vi "LINC Register COSMOS Commands.vi"(8 "error in":errorcluster, 11 "LINC session":refnum<class "LINC.lvclass">) -> (0 "error out":errorcluster, 3 "dup LINC session":refnum<class "LINC.lvclass">)   [LabVIEW 2018, in "STEPkgDriver_LINC.lvlib" / "LINC.lvclass"]
uses:
  LINC.lvclass
panel:
  in  "common commands":T1
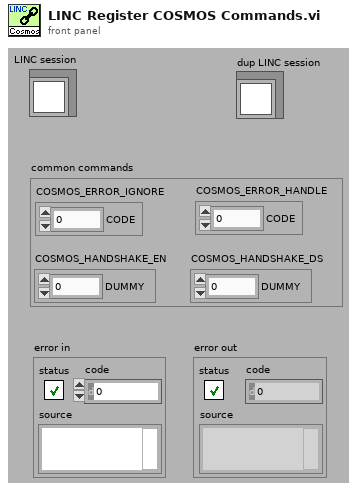
[diagram p1: front panel]
types:
  T1 = cluster{"COSMOS_ERROR_IGNORE":cluster{"CODE":i32}, "COSMOS_ERROR_HANDLE":cluster{"CODE":i32}, "COSMOS_HANDSHAKE_EN":cluster{"DUMMY":u8}, "COSMOS_HANDSHAKE_DS":cluster{"DUMMY":u8}}
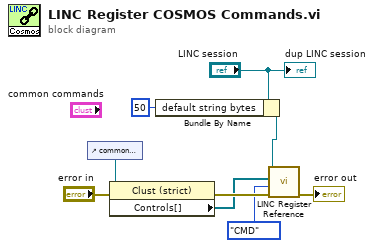
[diagram p0: block diagram]
diagram:
  n1 = control-ref of="common commands"() -> (w8:refnum<vi>)
  n2 = property class="Clust (strict)"(reference=w8, error in="error in") -> (error out=w7:errorcluster, "Controls[]"=w6:refnum<vi>[])  [unwired: 1 out]
  n3 = Bundle By Name(cluster="LINC session", "default string bytes"=50) -> (w2:refnum<class "LINC.lvclass">)
  n4 = call "LINC Register Reference.vi"("error in (no error)"=w7, "type (CMD)"=enum16{"CMD", "TLM", "CMD_HDR", "TLM_HDR"}."CMD", "controls"=w6, "LINC session"=w2) -> ("error out"=→"error out":errorcluster)  [unwired: 6 in, 1 out]
  "dup LINC session" <- "LINC session"
